vi "PicoHarp.vi"() -> ()   [LabVIEW 2019]
uses:
  phlib.dll
panel:
  in  "Acq.Time":i32=1000 min=1 max=3600000 step=100
  in  "Binning":i32 min=0 max=7 step=1
  out "Error":bool
  in  "Ch1 ZeroX":i32=10 min=0 max=20 step=1
  in  "Ch1 Level":i32=50 min=0 max=800 step=10
  in  "Ch0 ZeroX":i32=10 min=0 max=20 step=1
  in  "Ch0 Level":i32=50 min=0 max=800 step=10
  in  "Syncdiv":enum16{"1", "2", "4", "8"}(ring)=enum."8"
  out "Ch1Rate":i32(slide) scale=0.01..100000000.0 scale format="%.0e"
  in  "Stop On Overflow":bool=TRUE
  out "Oveflow":bool
  out "DLL Version (must be 3.0)":string caption="DLL Version"
  out "SyncRate":i32(slide) scale=0.01..100000000.0 scale format="%.0e"
  out "IntegralCount":i32
  out "Histogram":u32[](graph)
  out "Resol. (ps)":i32 min=0 max=2000 step=1
  out "Calibration Status":string
  in  "Run":bool
  in  "done":bool
  out "Initialization Status":string
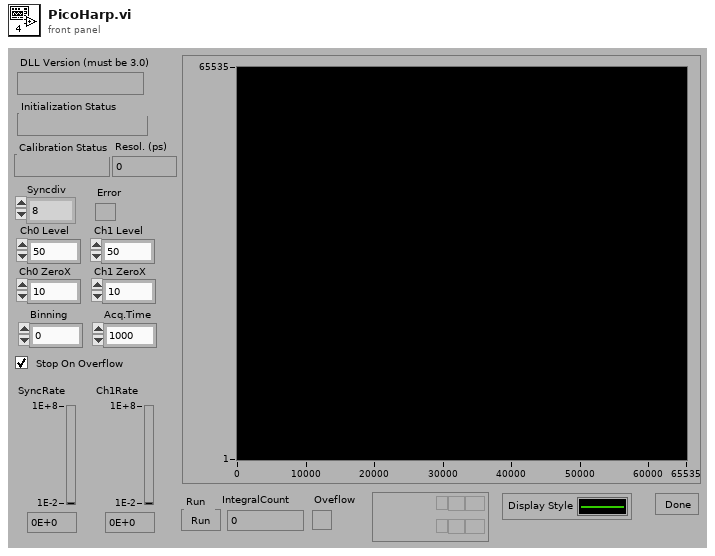
[diagram p1: front panel]
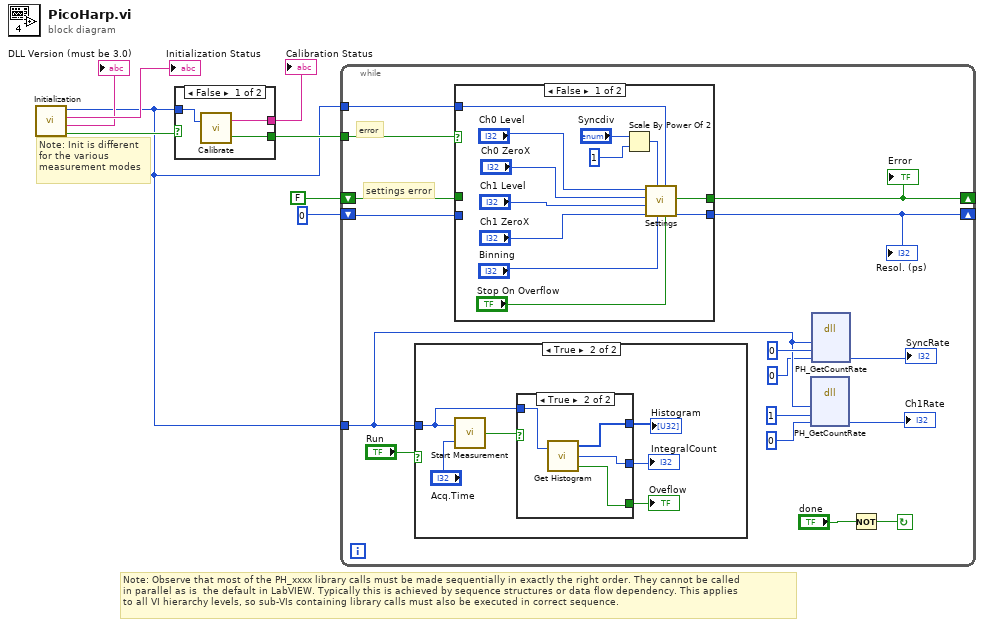
[diagram p0: block diagram]
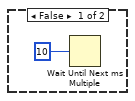
[diagram p2: hidden frame]
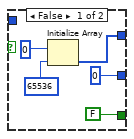
[diagram p3: hidden frame]
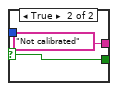
[diagram p5: hidden frame]
diagram:
  # "Note: Init is different \nfor the various\nmeasurement modes"
  # "Note: Observe that most of the PH_xxxx library calls must be made sequentially in exactly the right order. They cannot be called \nin parallel as is  the default in LabVIEW. Typically this is achieved by sequence structures or data flow dependency. This applies\nto all VI hierarchy levels, so sub-VIs containing library calls must also be executed in correct sequence."
  n1 = call "Initialization.vi"() -> ("Deviceindex"=w1:i32, "Initialization Status"=→"Initialization Status":string, "DLL Version"=→"DLL Version (must be 3.0)":string, "Initialization Error"=w4:bool)  [unwired: 2 in]
  n2 = case shown="False" w4 {
    selector: w4 -> [_ w12]
    tunnel: [w11 "Not calibrated"] -> w8
    tunnel: [w10 w12] -> w6
    tunnel: w1 -> [w9 _]
    frame False {
      n3 = call "Calibrate.vi"("Deviceindex"=w9) -> ("Calib Error"=w10:bool, "Status"=w11:string)  [unwired: 1 in]
    }
    frame True {
    }
  }
  "Calibration Status" <- w8
  n4 = while {
    tunnel: w1 -> [w19]
    tunnel: w1 -> [w21]
    tunnel: w6 -> [w25]
    shift-left: 0 -> [w26]
    shift-right: [w27] -> _
    shift-left: FALSE -> [w24]
    shift-right: [w22] -> _
    stop <- w28 continue-if-true
    # "settings error"
    # "error"
    n5 = case shown="True" "Run" {
      tunnel: w19 -> [_ w31]
      frame False {
        n6 = Wait Until Next ms Multiple(millisecond multiple=10) -> ()  [unwired: 1 out]
      }
      frame True {
        n7 = call "Start Measurement.vi"("Acquisition time"="Acq.Time", "DeviceIndex"=w31) -> ("DataValid"=w36:bool)
        n8 = case shown="True" w36 {
          tunnel: [w40 w45] -> w35
          tunnel: [FALSE w43] -> w33
          tunnel: [u32 0 w44] -> w34
          tunnel: w31 -> [_ w42]
          frame False {
            n9 = Initialize Array "Initialize Array"(u32 0, 65536) -> (w40:u32[])
          }
          frame True {
            n10 = call "Get Histogram.vi"("DeviceIndex"=w42) -> ("Histogram"=w45:u32[], "IntegralCount"=w44:i32, "Overflow"=w43:bool)  [unwired: 1 in]
          }
        }
        "Histogram" <- w35
        "IntegralCount" <- w34
        "Oveflow" <- w33
      }
    }
    n11 = case shown="False" w25 {
      tunnel: [w54 w59] -> w22
      tunnel: w24 -> [_ w59]
      tunnel: [w53 w58] -> w27
      tunnel: w26 -> [_ w58]
      tunnel: w21 -> [w46 _]
      frame False {
        n12 = Scale By Power Of 2(n="Syncdiv", x=1) -> (x*2^n=w48:i32)
        n13 = call "Settings.vi"("StopOnOverflow"="Stop On Overflow", "DeviceIndex"=w46, "Range No."="Binning", "SyncDiv"=w48, "CFD1 zero X"="Ch1 ZeroX", "CFD1 level"="Ch1 Level", "CFD0 zero X"="Ch0 ZeroX", "CFD0 level"="Ch0 Level") -> ("Resolution"=w53:i32, "Error"=w54:bool)  [unwired: 2 in]
      }
      frame True {
      }
    }
    "Resol. (ps)" <- w27
    "Error" <- w22
    n14 = dll-call lib="phlib.dll" fn="PH_GetCountRate"("devidx"=w19, "channel"=1, "rate"=0) -> ("rate"=→"Ch1Rate":i32)  [unwired: 6 in, 2 out]
    n15 = dll-call lib="phlib.dll" fn="PH_GetCountRate"("devidx"=w19, "channel"=0, "rate"=0) -> ("rate"=→"SyncRate":i32)  [unwired: 6 in, 2 out]
    n16 = Not(x="done") -> (.not. x?=w28:bool)
  }
